vi "RS_FF.vi"(8 "Set":bool, 10 "Reset":bool) -> (2 "Result":bool)   [LabVIEW 2010, in "kevLib2011.lvlib"]
uses:
  kevLib2011.lvlib
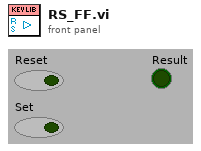
[diagram p1: front panel]
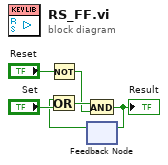
[diagram p0: block diagram]
diagram:
  n1 = Not(x="Reset") -> (.not. x?=w5:bool)
  n2 = feedback #1() -> (w1:bool)  [unwired: 1 out]
  n3 = Or(x=w1, y="Set") -> (x .or. y?=w6:bool)
  n4 = And(x=w6, y=w5) -> (x .and. y?=w2:bool)
  "Result" <- w2
  n5 = feedback-in #1(w2) -> ()
